vi "Hurt By Wall.vi"(9 "Array":i32[][](array[numeric]), 10 "Map Length":i32, 11 "Map  Width":i32) -> (3 "Boolean":bool)   [LabVIEW 2014]
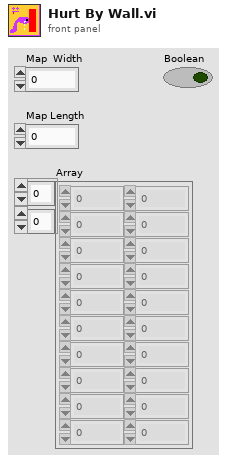
[diagram p1: front panel]
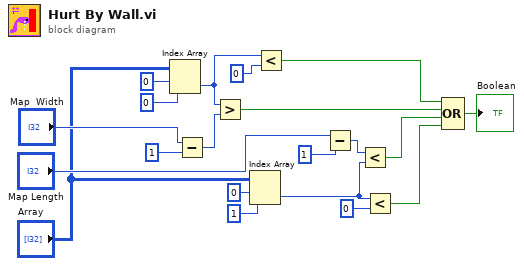
[diagram p0: block diagram]
diagram:
  n1 = Index Array(array="Array", index (row)=0, index (col)=0 ("disabled index (col)")) -> (element=w7:i32)
  n2 = Subtract(x="Map  Width", y=1) -> (x-y=w6:i32)
  n3 = Greater?(x=w7, y=w6) -> (0:w14:bool)
  n4 = Index Array(array="Array", index (row)=0, index (col)=1 ("disabled index (col)")) -> (element=w11:i32)
  n5 = Less?(x=w7, y=0) -> (x < y?=w13:bool)
  n6 = Subtract(x="Map Length", y=1) -> (x-y=w10:i32)
  n7 = Less?(x=w10, y=w11) -> (x < y?=w15:bool)
  n8 = Less?(x=w11, y=0) -> (x < y?=w16:bool)
  n9 = Compound Arithmetic op=OR(w13, w14, w15, w16) -> (→"Boolean":bool)
